vi "Is_Amount_Enough.vi"(0 "Vending_data":T1) -> (4 "Is_Amount_Enough?":bool, 8 "Total_Amount":dbl)   [LabVIEW 2023]
uses:
  Controls/Vending_Data.ctl
  Controls/Total_Cash_Count.ctl
  Controls/Inserted_Cash_Count.ctl
  Controls/Drink_Quantity.ctl
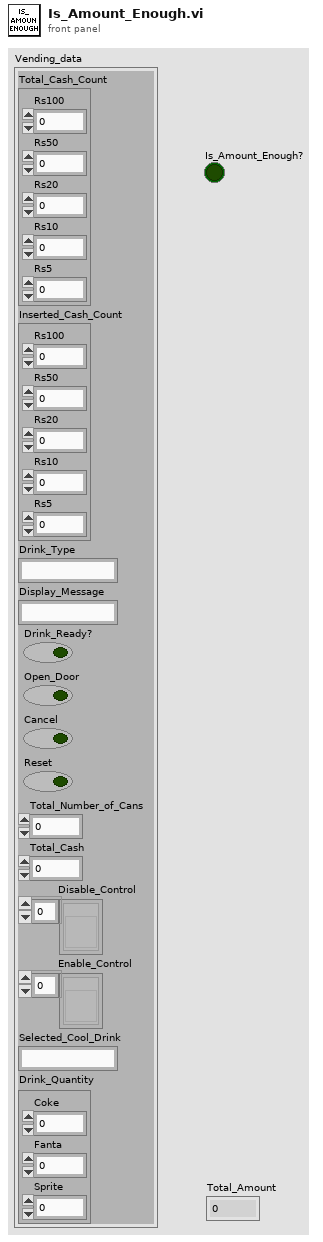
[diagram p1: front panel]
types:
  T1 = typedef "Vending_Data.ctl" = cluster{"Total_Cash_Count":T2, "Inserted_Cash_Count":T3, "Drink_Type":string, "Display_Message":string, "Drink_Ready?":bool, "Open_Door":bool, "Cancel":bool, "Reset":bool, "Total_Number_of_Cans":i32, "Total_Cash":i32, "Disable_Control":refnum<vi>[], "Enable_Control":refnum<vi>[], "Selected_Cool_Drink":string, "Drink_Quantity":T4}
  T2 = typedef "Total_Cash_Count.ctl" = cluster{"Rs100":i32, "Rs50":i32, "Rs20":i32, "Rs10":i32, "Rs5":i32}
  T3 = typedef "Inserted_Cash_Count.ctl" = cluster{"Rs100":i32, "Rs50":i32, "Rs20":i32, "Rs10":i32, "Rs5":i32}
  T4 = typedef "Drink_Quantity.ctl" = cluster{"Coke":dbl, "Fanta":dbl, "Sprite":dbl}
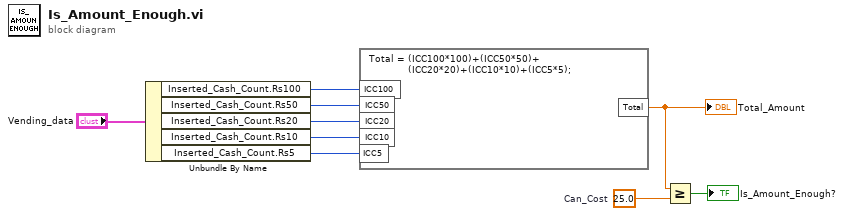
[diagram p0: block diagram]
diagram:
  w9 = 25.0  # Can_Cost
  n1 = Unbundle By Name("Vending_data") -> ("Inserted_Cash_Count.Rs100"=w3:i32, "Inserted_Cash_Count.Rs50"=w4:i32, "Inserted_Cash_Count.Rs20"=w5:i32, "Inserted_Cash_Count.Rs10"=w6:i32, "Inserted_Cash_Count.Rs5"=w7:i32)
  n2 = formula code="Total = (ICC100*100)+(ICC50*50)+\n             (ICC20*20)+(ICC10*10)+(ICC5*5);"("ICC100"=w3, "ICC50"=w4, "ICC20"=w5, "ICC10"=w6, "ICC5"=w7) -> ("Total"=w8:dbl)
  "Total_Amount" <- w8
  n3 = Greater Or Equal?(x=w8, y=w9) -> (x >= y?=→"Is_Amount_Enough?":bool)
